vi "RFIDWrite.vi"(0 "Device In":u64, 5 "string":string caption="Tag String", 7 "protocol":i32(ring) caption="Protocol" items=["PROTOCOL_EM4100"=1, "PROTOCOL_ISO11785_FDX_B"=2, "PROTOCOL_PHIDGETS"=3], 9 "Lock":bool caption="Lock Tag", 11 "error in (no error)":errorcluster) -> (4 "Device Out":u64, 15 "error out":errorcluster)   [LabVIEW 2012, in "Phidget RFID.lvlib"]
doc: "${Write:Header}"
uses:
  <instrlib>/Phidgets/Phidget RFID/Phidget RFID.lvlib
  <instrlib>/Phidgets/Phidget Common/Phidget Common.lvlib
  phidget22.dll
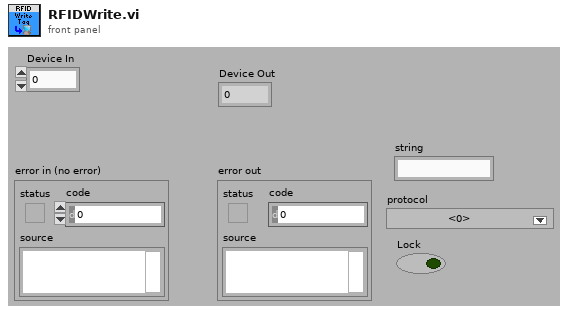
[diagram p1: front panel]
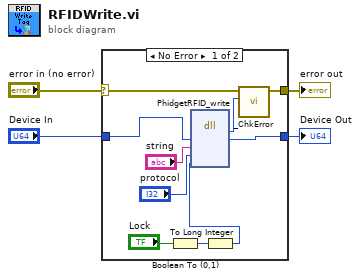
[diagram p0: block diagram]
diagram:
  n1 = case shown="No Error" "error in (no error)" {
    selector: "error in (no error)" -> [w12 w16]
    tunnel: [w11 w16] -> w3
    tunnel: "Device In" -> [w14 w15]
    tunnel: [w13 w15] -> w1
    frame No Error {
      n2 = Boolean To (0,1)(Boolean="Lock") -> (0, 1=w7:i16)
      n3 = To Long Integer(number=w7) -> (32bit integer=w5:i32)
      n4 = dll-call lib="phidget22.*" fn="PhidgetRFID_write" ("phidget21.*:CPhidgetTextLCD_setDisplayString")("phid"=w14, "str"="string", "protocol"="protocol", "lock"=w5) -> ("return type"=w10:i32, "phid"=w13:u64)  [unwired: 6 in, 2 out]
      n5 = call <instrlib>:"_ChkError.vi"("Return Code"=w10, "error in (no error)"=w12) -> ("error out"=w11:errorcluster)  [unwired: 9 in]
    }
    frame Error {
    }
  }
  "error out" <- w3
  "Device Out" <- w1
